vi "Test of the NRP-Z2X class.vi"() -> ()   [LabVIEW 2020, in "RS Z2X.lvclass"]
uses:
  RS Z2X.lvclass
  C:/Sandbox/Git_Sandbox/WiSpry Test Framework source code (LV20)/WiSpry Test Framework/Instruments/Instrument.lvclass
  Instrument.lvclass/Instrument.ctl
  Instrument.lvclass
panel:
  out "Power Out":dbl
  in  "Frequency":dbl
  in  "VISA resource name":refnum<visa-resource-name>
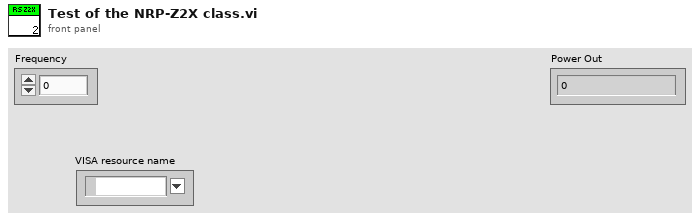
[diagram p1: front panel]
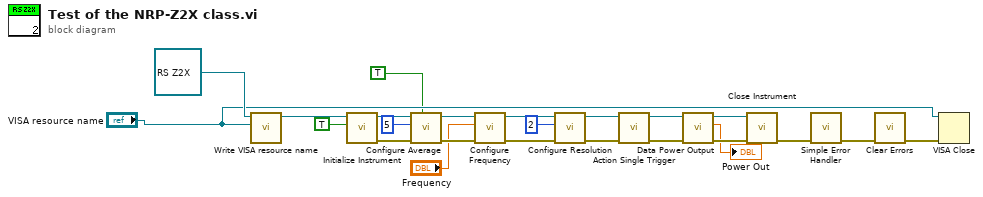
[diagram p0: block diagram]
diagram:
  n1 = call "Write VISA resource name.vi"("VISA resource name"="VISA resource name", "Instrument in"=refnum<class "RS Z2X.lvclass"> refnum ("RS Z2X.lvclass")) -> ("Instrument out"=w23:refnum<class "RS Z2X.lvclass">)  [unwired: 9 in]
  n2 = call-dynamic "Initialize Instrument.vi"("Reset"=TRUE, "RS Z2X in"=w23) -> ("error out"=w19:errorcluster, "RS Z2X out"=w18:refnum<class "RS Z2X.lvclass">)  [unwired: 8 in]
  n3 = call-dynamic "Configure Average.vi"("Average on"=TRUE, "error in (no error)"=w19, "Average Count"=5, "RS Z2X in"=w18) -> ("error out"=w15:errorcluster, "RS Z2X out"=w14:refnum<class "RS Z2X.lvclass">)  [unwired: 6 in]
  n4 = call-dynamic "Configure Frequency.vi"("error in (no error)"=w15, "Frequency"="Frequency", "RS Z2X in"=w14) -> ("error out"=w12:errorcluster, "RS Z2X out"=w11:refnum<class "RS Z2X.lvclass">)  [unwired: 7 in]
  n5 = call-dynamic "Configure Resolution.vi"("error in (no error)"=w12, "Resolution"=2, "RS Z2X in"=w11) -> ("error out"=w9:errorcluster, "RS Z2X out"=w8:refnum<class "RS Z2X.lvclass">)  [unwired: 7 in]
  n6 = call-dynamic "Action Single Trigger.vi"("error in (no error)"=w9, "RS Z2X in"=w8) -> ("error out"=w7:errorcluster, "RS Z2X out"=w6:refnum<class "RS Z2X.lvclass">)  [unwired: 8 in]
  n7 = call-dynamic "Data Power Output.vi"("error in (no error)"=w7, "RS Z2X in"=w6) -> ("error out"=w5:errorcluster, "Power Out"=→"Power Out":dbl, "RS Z2X out"=w4:refnum<class "RS Z2X.lvclass">)  [unwired: 7 in]
  n8 = call-dynamic "Close Instrument.vi"("error in (no error)"=w5, "Instrument in"=w4) -> ("error out"=w3:errorcluster)  [unwired: 8 in, 1 out]
  n9 = call <vilib>:"Simple Error Handler.vi"("error in (no error)"=w3) -> ("error out"=w2:errorcluster)  [unwired: 4 in, 4 out]
  n10 = call <vilib>:"Clear Errors.vi"("error in (no error)"=w2) -> ("error out"=w22:errorcluster)  [unwired: 5 in, 1 out]
  n11 = VISA Close(VISA resource name="VISA resource name", error in (no error)=w22) -> ()  [unwired: 1 out]
